vi "aw_WRDCluster_8acel_FALLOS_SUBIDA.vi"(0 "Array TAGs":string[](array[string]), 1 "Max RMS Ruedas":dbl[][](array[numeric]), 2 "TimeStamp":dbl, 3 "p_sp":dbl, 4 "p_tp":dbl) -> (6 "JSON cluster":T1)   [LabVIEW 2015]
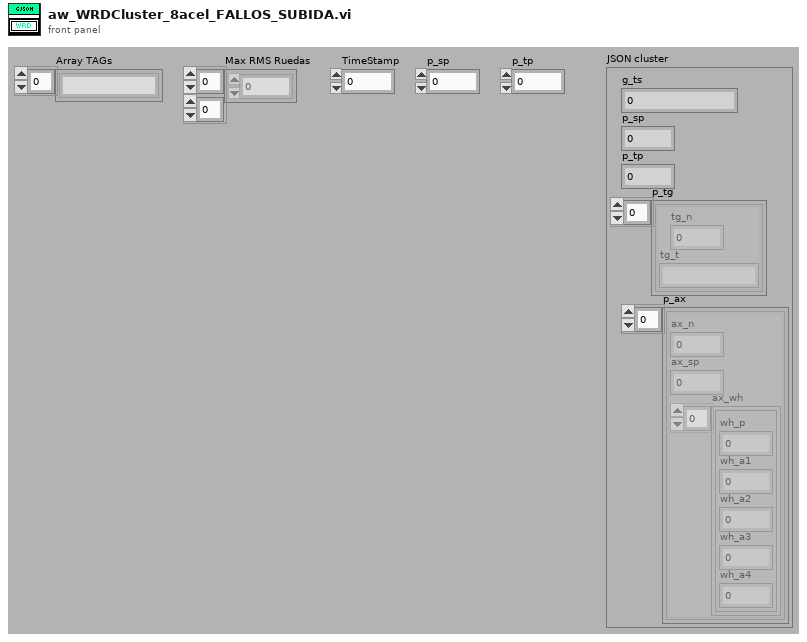
[diagram p1: front panel]
types:
  T1 = cluster{"g_ts":dbl, "p_sp":dbl, "p_tp":dbl, "p_tg":cluster{"tg_n":dbl, "tg_t":string}[], "p_ax":cluster{"ax_n":dbl, "ax_sp":dbl, "ax_wh":cluster{"wh_p":dbl, "wh_a1":dbl, "wh_a2":dbl, "wh_a3":dbl, "wh_a4":dbl}[]}[]}
  T2 = cluster{"wh_p":dbl, "wh_a1":dbl, "wh_a2":dbl, "wh_a3":dbl, "wh_a4":dbl}
  T3 = cluster{"ax_n":dbl, "ax_sp":dbl, "ax_wh":cluster{"wh_p":dbl, "wh_a1":dbl, "wh_a2":dbl, "wh_a3":dbl, "wh_a4":dbl}[]}
  T4 = cluster{"wh_p":dbl, "wh_a1":dbl, "wh_a2":dbl, "wh_a3":dbl, "wh_a4":dbl}[]
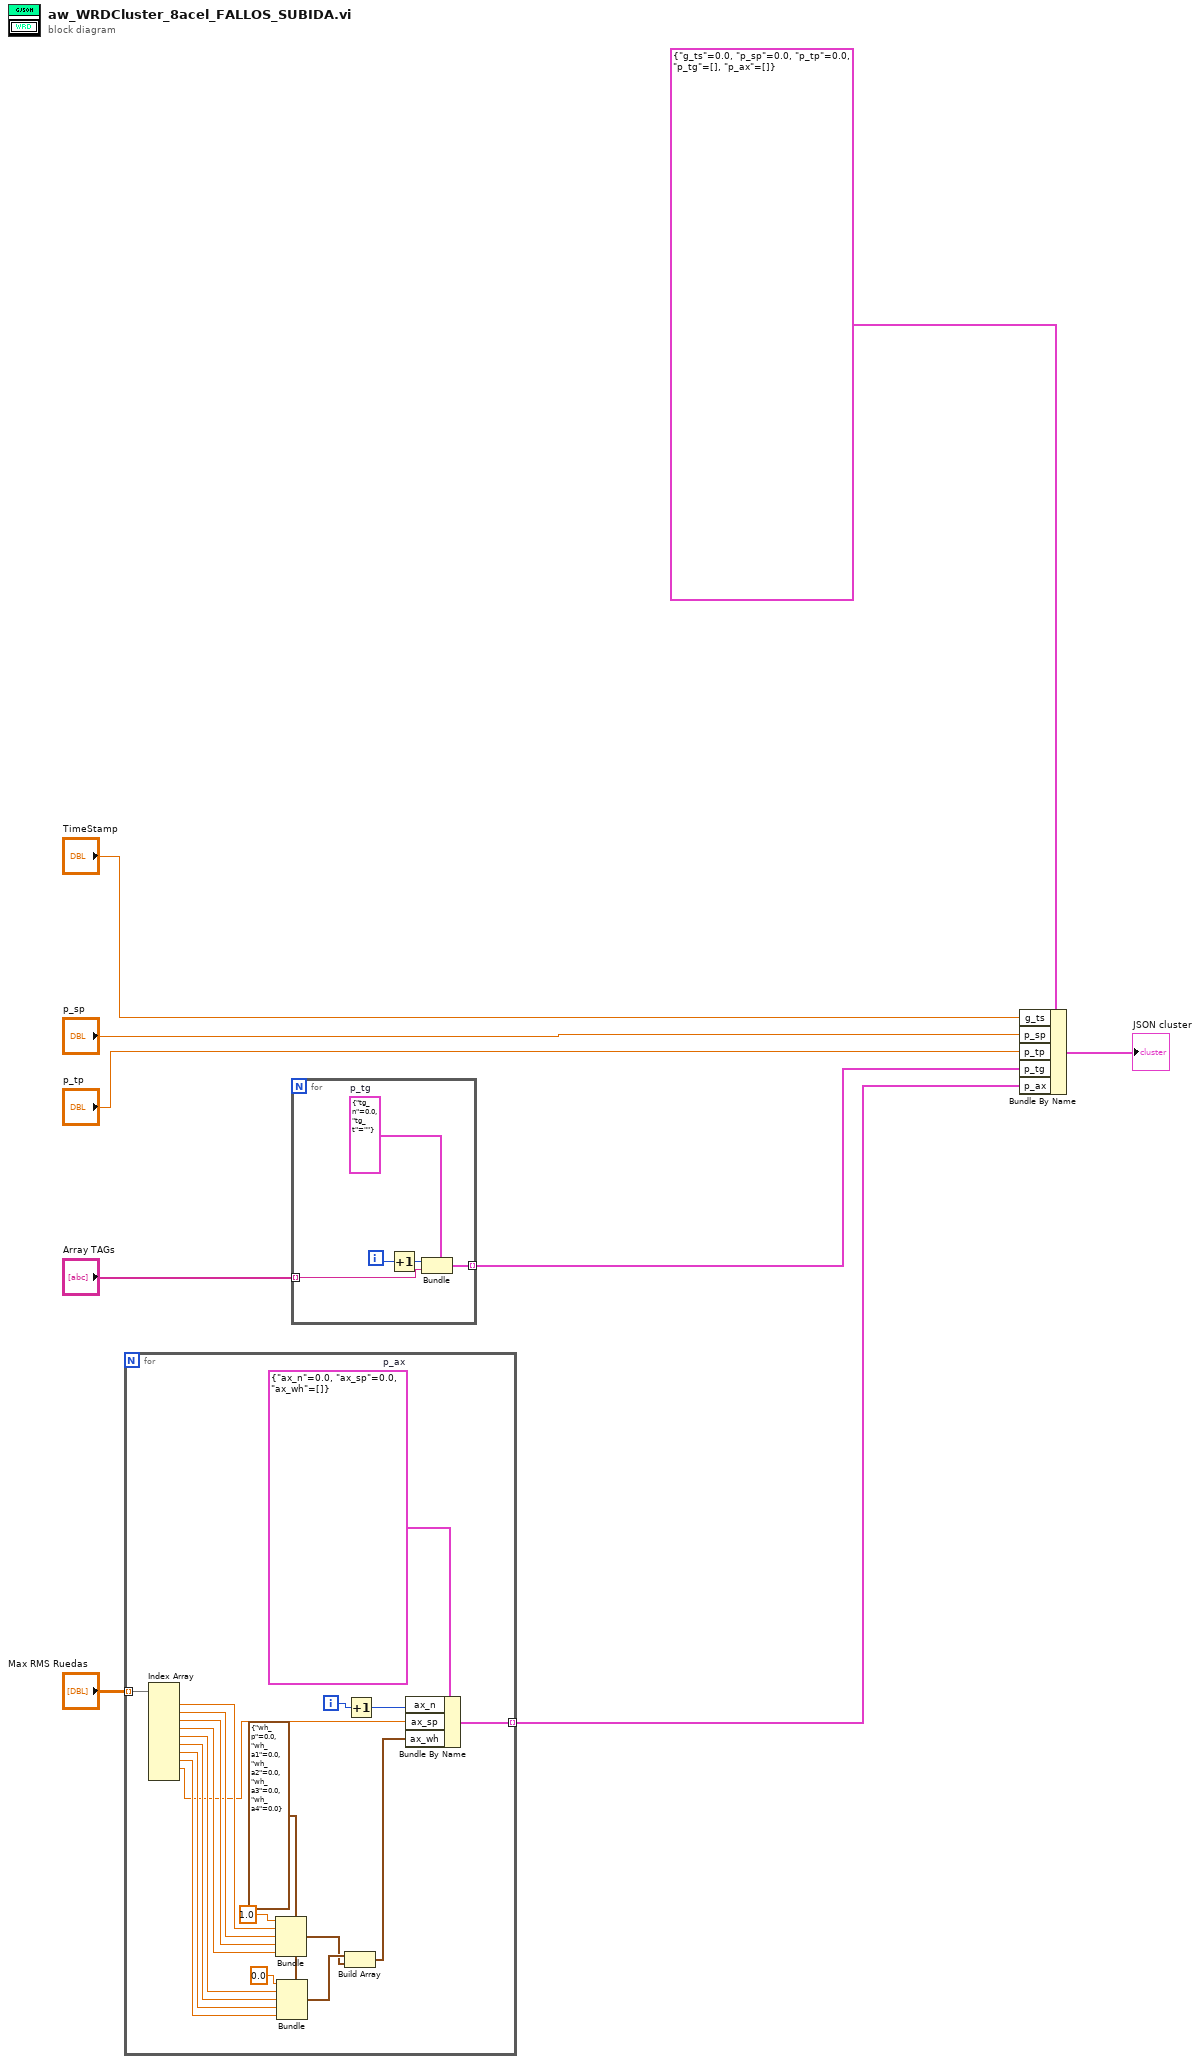
[diagram p0: block diagram]
diagram:
  n1 = for {
    tunnel: "Max RMS Ruedas" -> [w29] mode=indexing
    tunnel: [w20] -> w3 mode=indexing
    i -> [w27]
    w19 = T2 {"wh_p"=0.0, "wh_a1"=0.0, "wh_a2"=0.0, "wh_a3"=0.0, "wh_a4"=0.0} ("ax_wh")
    w28 = T3 {"ax_n"=0.0, "ax_sp"=0.0, "ax_wh"=[]}  # p_ax
    n2 = Index Array(array=w29) -> (element #1=w24:dbl, element #2=w22:dbl, element #3=w16:dbl, element #4=w15:dbl, element #5=w14:dbl, element #6=w13:dbl, element #7=w12:dbl, element #8=w11:dbl, element #9=w10:dbl)  [unwired: 10 in, 1 out]
    n3 = Bundle(cluster=w19, "wh_p"=1.0, "wh_a1"=w24, "wh_a2"=w22, "wh_a3"=w16, "wh_a4"=w15) -> (w17:T2)
    n4 = Bundle(cluster=w19, "wh_p"=0.0, "wh_a1"=w14, "wh_a2"=w13, "wh_a3"=w12, "wh_a4"=w11) -> (w18:T2)
    n5 = Build Array(w18, w17) -> (w21:T4)
    n6 = Increment(x=w27) -> (x+1=w26:i32)
    n7 = Bundle By Name(cluster=w28, "ax_n"=w26, "ax_sp"=w10, "ax_wh"=w21) -> (w20:T3)
  }
  n8 = for {
    tunnel: "Array TAGs" -> [w31] mode=indexing
    tunnel: [w30] -> w8 mode=indexing
    i -> [w32]
    w34 = cluster{"tg_n":dbl, "tg_t":string} {"tg_n"=0.0, "tg_t"=""}  # p_tg
    n9 = Increment(x=w32) -> (x+1=w33:i32)
    n10 = Bundle(cluster=w34, "tg_n"=w33, "tg_t"=w31) -> (w30:cluster{"tg_n":dbl, "tg_t":string})
  }
  n11 = Bundle By Name(cluster=T1 {"g_ts"=0.0, "p_sp"=0.0, "p_tp"=0.0, "p_tg"=[], "p_ax"=[]}, "g_ts"="TimeStamp", "p_sp"="p_sp", "p_tp"="p_tp", "p_tg"=w8, "p_ax"=w3) -> (→"JSON cluster":T1)
